vi "Sub_vi_ejecutar_Edificio_3.vi"(0 "Edificio_string":string, 1 "Serv_Numeric":u8, 2 "De":u8=1 min=1 max=16, 3 "Hasta":u8=16 min=1 max=16, 4 "edo_actual_aula":bool, 5 "rango":bool, 6 "+                 -":bool) -> ()   [LabVIEW 2017]
uses:
  GlobalFag.vi
  Global_comSerie.vi
  <vilib>/Instr/_visa.llb/VISA Configure Serial Port (Instr).vi
panel:
  in  "x":u8
  out "sh_reg2":u8
  out "sh_reg":u8
  in  "act_vac":bool
  out "estado 2":bool[](array[boolean])
  out "aula_fin":u8
  in  "stop_edificio":bool
  in  "Servicios":bool[](array[boolean])
  # "+/- Edo. Actual"
  # "Conf para Edif A, aula 15"
  # "Servicio"
  # "Aplicar a un rango"
  # "Luz"
  # "Aire"
  # "Proyector"
  # "Agua"
  # "Acceso"
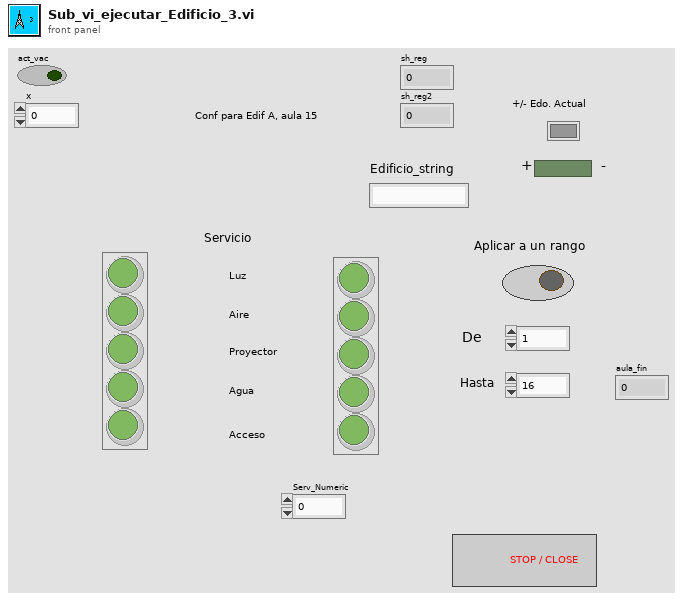
[diagram p1: front panel]
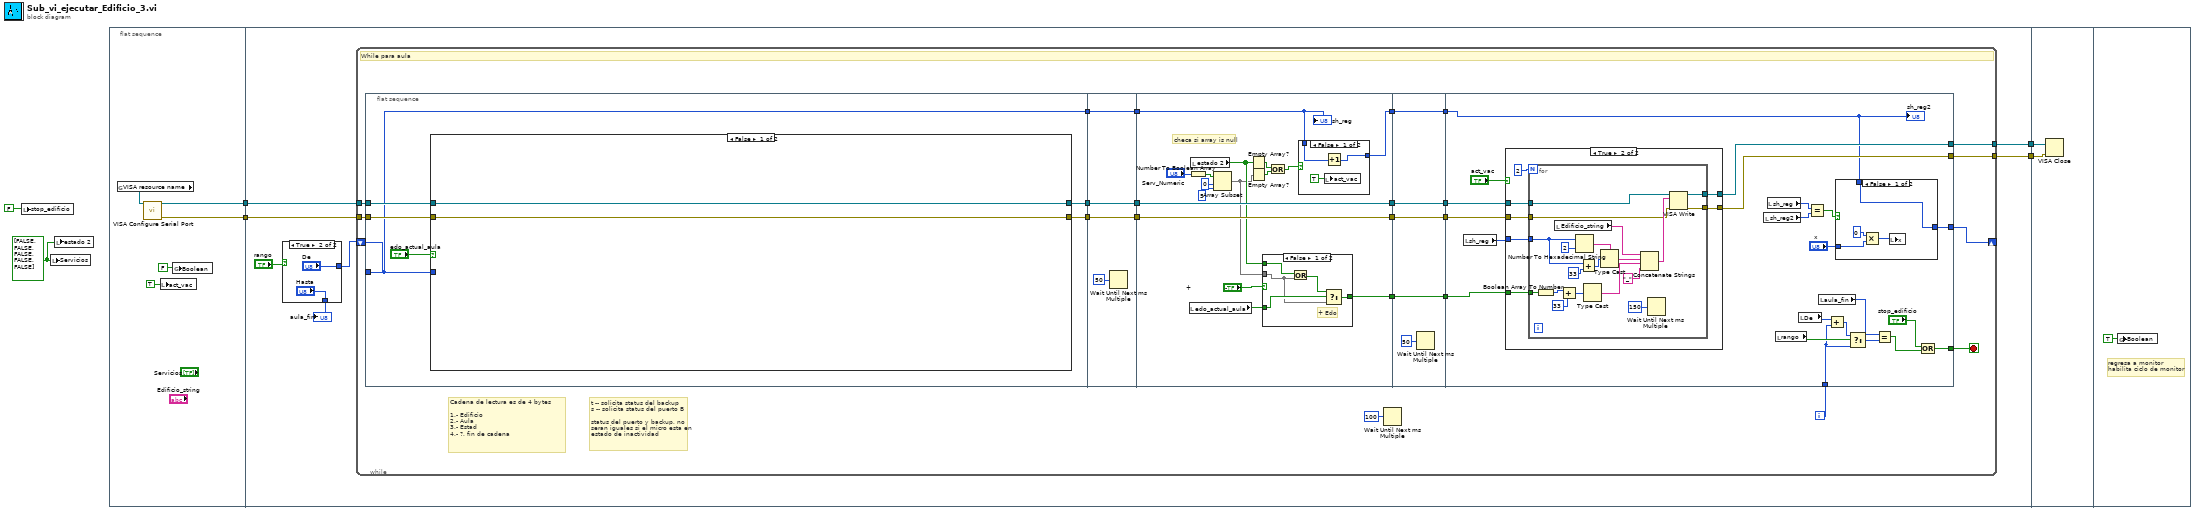
[diagram p0: block diagram]
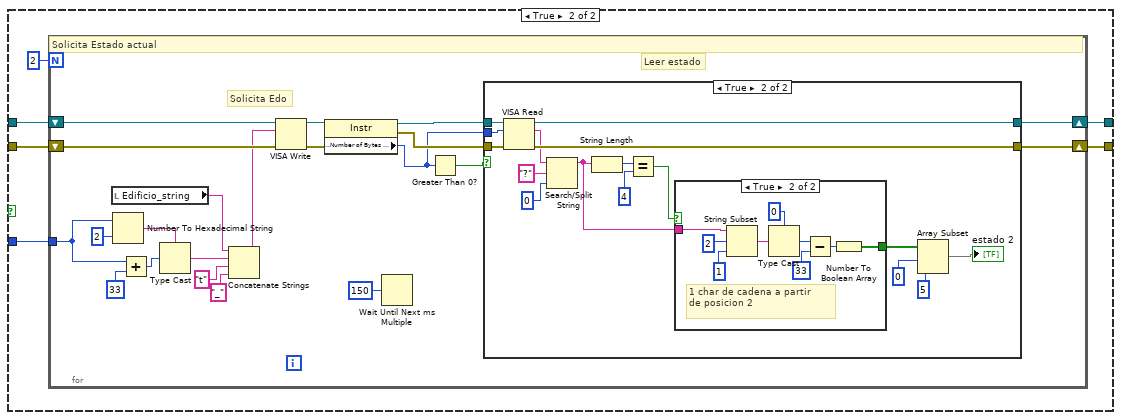
[diagram p2: hidden frame]
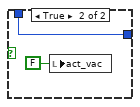
[diagram p5: hidden frame]
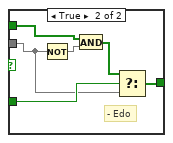
[diagram p6: hidden frame]
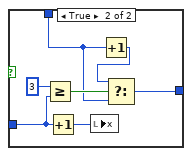
[diagram p7: hidden frame]
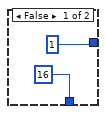
[diagram p9: hidden frame]
diagram:
  w1 = bool[] [FALSE, FALSE, FALSE, FALSE, FALSE] ("Servicios")
  n1 = local write "stop_edificio"(FALSE ("Loading")) -> ()
  n2 = local write "Servicios"(w1) -> ()
  n3 = local write "estado 2"(w1) -> ()
  n4 = flat-sequence {
    tunnel: [w11] -> w5
    tunnel: [w10] -> w4
    tunnel: w4 -> [w15]
    tunnel: w5 -> [w16]
    tunnel: [w13] -> w3
    tunnel: [w12] -> w2
    tunnel: w3 -> [w211]
    tunnel: w2 -> [w210]
    frame #0 {
      n5 = global read "Global_comSerie.vi" "VISA resource name"() -> (w8:refnum<visa-resource-name>)
      n6 = call-poly "VISA Configure Serial Port"("VISA resource name"=w8) -> ("VISA resource name out"=w11:refnum<visa-resource-name>, "error out"=w10:errorcluster)  [unwired: 13 in]
      n7 = local write "act_vac"(TRUE ("act_vac")) -> ()
      n8 = global write "GlobalFag.vi" "Boolean"(FALSE ("Boolean")) -> ()
    }
    frame #1 {
      n9 = case shown="True" "rango" {
        tunnel: [u8 1 ("width (-)") "De"] -> w14
        tunnel: [u8 16 ("width (-)") "Hasta"] -> w17
        frame False {
        }
        frame True {
        }
      }
      "aula_fin" <- w17
      n10 = while {
        shift-right: [w21] -> _
        shift-left: w14 -> [w40]
        tunnel: w16 -> [w39]
        tunnel: w15 -> [w38]
        tunnel: [w23] -> w13
        tunnel: [w22] -> w12
        i -> [w19]
        stop <- w20 stop-if-true
        # "Cadena de lectura es de 4 bytes\n\n1.- Edificio\n2.- Aula\n3.- Estad\n4.- ?, fin de cadena"
        # "t -- solicita status del backup\ns -- solicita status del puerto B\n\nstatus del puerto y backup, no \nseran iguales si el micro esta en\nestado de inactividad"
        # "While para aula"
        n11 = flat-sequence {
          tunnel: w40 -> [w44]
          tunnel: w39 -> [w46]
          tunnel: w38 -> [w45]
          tunnel: [w44] -> w37
          tunnel: [w43] -> w35
          tunnel: [w42] -> w33
          tunnel: w37 -> [w107]
          tunnel: [w107] -> w36
          tunnel: w35 -> [w106]
          tunnel: [w106] -> w34
          tunnel: w33 -> [w105]
          tunnel: [w105] -> w32
          tunnel: [w112] -> w31
          tunnel: w36 -> [w111]
          tunnel: [w122] -> w29
          tunnel: [w121] -> w27
          tunnel: w34 -> [w121]
          tunnel: [w120] -> w25
          tunnel: w32 -> [w120]
          tunnel: w31 -> [w144]
          tunnel: [w144] -> w30
          tunnel: w29 -> [w143]
          tunnel: [w143] -> w28
          tunnel: w27 -> [w142]
          tunnel: [w142] -> w26
          tunnel: w25 -> [w141]
          tunnel: [w141] -> w24
          tunnel: w30 -> [w155]
          tunnel: w28 -> [w164]
          tunnel: w26 -> [w166]
          tunnel: w24 -> [w165]
          tunnel: [w161] -> w23
          tunnel: [w160] -> w22
          tunnel: [w154] -> w21
          tunnel: [w146] -> w20
          tunnel: w19 -> [w145]
          frame #0 {
            n12 = case shown="False" "edo_actual_aula" {
              tunnel: w44 -> [_ w54]
              tunnel: w46 -> [w49 w53]
              tunnel: w45 -> [w48 w52]
              tunnel: [w49 w51] -> w43
              tunnel: [w48 w50] -> w42
              frame False {
              }
              frame True {
                n13 = for {
                  N: 2 -> [_]
                  tunnel: w54 -> [w58]
                  shift-right: [w74] -> w51
                  shift-left: w53 -> [w72]
                  shift-right: [w73] -> w50
                  shift-left: w52 -> [w71]
                  # "Solicita Edo"
                  # "Leer estado"
                  # "Solicita Estado actual"
                  n14 = local read "Edificio_string"() -> (w56:string)
                  n15 = Number To Hexadecimal String(1:u8 2 ("width (-)"), 2:w58) -> (0:w60:string)
                  n16 = Add(x=w58, y=u8 33 ("width (-)")) -> (x+y=w62:u8)
                  n17 = Type Cast(type=w60, x=w62) -> (*(type *) &x=w57:string)
                  n18 = Concatenate Strings(w56, w57, "t" ("string"), "_" ("string")) -> (w70:string)
                  n19 = VISA Write(VISA resource name=w72, write buffer=w70, error in (no error)=w71) -> (VISA resource name out=w75:refnum<visa-resource-name>, error out=w76:errorcluster)  [unwired: 1 out]
                  n20 = property class="Instr"(reference=w75, error in=w76) -> (reference out=w65:refnum<visa-resource-name>, error out=w64:errorcluster, "Serial Settings:Number of Bytes at Serial Port"=w63:u32)
                  n21 = Wait Until Next ms Multiple(millisecond multiple=u32 150) -> ()  [unwired: 1 out]
                  n22 = Greater Than 0?(x=w63) -> (x > 0?=w66:bool)
                  n23 = case shown="True" w66 {
                    tunnel: w65 -> [w77 w94]
                    tunnel: w64 -> [w78 w93]
                    tunnel: [w78 w92] -> w73
                    tunnel: [w77 w91] -> w74
                    tunnel: w63 -> [_ w90]
                    frame False {
                    }
                    frame True {
                      n24 = VISA Read(VISA resource name=w94, byte count=w90, error in (no error)=w93) -> (VISA resource name out=w91:refnum<visa-resource-name>, read buffer=w86:string, error out=w92:errorcluster)  [unwired: 1 out]
                      n25 = Search/Split String(string=w86, search string/char (-)="?", offset (0)=u8 0) -> (substring before match=w84:string)  [unwired: 2 out]
                      n26 = String Length(string=w84) -> (length=w89:i32)
                      n27 = Equal?(x=w89, y=4) -> (x = y?=w85:bool)
                      n28 = case shown="True" w85 {
                        tunnel: w84 -> [_ w96]
                        tunnel: [_ w95] -> w81
                        frame False {
                        }
                        frame True {
                          # "1 char de cadena a partir \nde posicion 2"
                          n29 = String Subset(string=w96, offset (0)=2, length (rest)=1 ("length (rest)")) -> (substring=w100:string)
                          n30 = Type Cast(type=u8 0 ("width (-)"), x=w100) -> (*(type *) &x=w98:u8)
                          n31 = Subtract(x=w98, y=u8 33) -> (x-y=w99:u8)
                          n32 = Number To Boolean Array(number=w99) -> (Boolean array=w95:bool[])
                        }
                      }
                      n33 = Array Subset(array=w81, index=0, length=5) -> (→"estado 2":bool[])
                    }
                  }
                }
              }
            }
          }
          frame #1 {
            n34 = Wait Until Next ms Multiple(millisecond multiple=u32 50) -> ()  [unwired: 1 out]
          }
          frame #2 {
            # "checa si array is null"
            n35 = local read "edo_actual_aula"() -> (w119:bool)
            n36 = Number To Boolean Array(number="Serv_Numeric") -> (Boolean array=w116:bool[])
            n37 = local read "estado 2"() -> (w110:bool[])
            n38 = Array Subset(array=w116, index=0, length=5) -> (w109:bool[])
            n39 = Empty Array?(array=w110) -> (empty?=w115:bool)
            n40 = Empty Array?(array=w109) -> (empty?=w114:bool)
            n41 = case shown="False" "+                 -" {
              tunnel: [w133 w139] -> w122
              tunnel: w119 -> [w131 w136]
              tunnel: w110 -> [w130 w135]
              tunnel: w109 -> [w129 w134]
              frame False {
                # "+ Edo"
                n42 = Or(x=w130, y=w129) -> (x .or. y?=w132:bool[])
                n43 = Select(t=w132, s=w131, f=w129) -> (s? t:f=w133:bool[])
              }
              frame True {
                # "- Edo"
                n44 = Not(x=w134) -> (.not. x?=w138:bool[])
                n45 = And(x=w135, y=w138) -> (x .and. y?=w137:bool[])
                n46 = Select(t=w137, s=w136, f=w134) -> (s? t:f=w139:bool[])
              }
            }
            n47 = Or(x=w115, y=w114) -> (x .or. y?=w113:bool)
            n48 = case shown="False" w113 {
              tunnel: [w125 w127] -> w112
              tunnel: w111 -> [w126 w127]
              frame False {
                n49 = local write "act_vac"(TRUE ("act_vac")) -> ()
                n50 = Increment(x=w126) -> (x+1=w125:u8)
              }
              frame True {
                n51 = local write "act_vac"(FALSE ("act_vac")) -> ()
              }
            }
            "sh_reg" <- w111
          }
          frame #3 {
            n52 = Wait Until Next ms Multiple(millisecond multiple=u32 50) -> ()  [unwired: 1 out]
          }
          frame #4 {
            n53 = local read "sh_reg"() -> (w162:u8)
            n54 = case shown="True" "act_vac" {
              tunnel: [w179 w186] -> w160
              tunnel: [w178 w185] -> w161
              tunnel: w162 -> [_ w184]
              tunnel: w166 -> [w178 w182]
              tunnel: w165 -> [w179 w181]
              tunnel: w164 -> [_ w180]
              frame False {
              }
              frame True {
                n55 = for {
                  N: 2 -> [_]
                  tunnel: [w194] -> w186
                  tunnel: [w193] -> w185
                  tunnel: w184 -> [w191]
                  tunnel: w180 -> [w190]
                  tunnel: w182 -> [w189]
                  tunnel: w181 -> [w188]
                  n56 = Boolean Array To Number(Boolean array=w190) -> (number=w192:u8)
                  n57 = local read "Edificio_string"() -> (w205:string)
                  n58 = Add(x=w192, y=u8 33) -> (x+y=w203:u8)
                  n59 = Number To Hexadecimal String(1:u8 2 ("width (-)"), 2:w191) -> (0:w200:string)
                  n60 = Add(x=w191, y=u8 33 ("width (-)")) -> (x+y=w202:u8)
                  n61 = Type Cast(x=w203) -> (*(type *) &x=w204:string)  [unwired: 1 in]
                  n62 = Type Cast(type=w200, x=w202) -> (*(type *) &x=w199:string)
                  n63 = Concatenate Strings(w205, w199, w204, "_" ("string")) -> (w201:string)
                  n64 = Wait Until Next ms Multiple(millisecond multiple=u32 150) -> ()  [unwired: 1 out]
                  n65 = VISA Write(VISA resource name=w189, write buffer=w201, error in (no error)=w188) -> (VISA resource name out=w193:refnum<visa-resource-name>, error out=w194:errorcluster)  [unwired: 1 out]
                }
              }
            }
            n66 = local read "sh_reg2"() -> (w158:u8)
            n67 = local read "sh_reg"() -> (w159:u8)
            n68 = local read "rango"() -> (w150:bool)
            n69 = local read "De"() -> (w152:u8)
            n70 = Equal?(x=w159, y=w158) -> (x = y?=w157:bool)
            n71 = local read "aula_fin"() -> (w149:u8)
            n72 = Add(x=w152, y=w145) -> (x+y=w151:i32)
            n73 = case shown="False" w157 {
              tunnel: "x" -> [w170 w176]
              tunnel: w155 -> [w167 w173]
              tunnel: [w167 w171] -> w154
              frame False {
                n74 = Multiply(x=u8 0, y=w170) -> (x*y=w168:u8)
                n75 = local write "x"(w168) -> ()
              }
              frame True {
                n76 = Greater Or Equal?(x=u8 3, y=w176) -> (x >= y?=w174:bool)
                n77 = Increment(x=w176) -> (x+1=w175:u8)
                n78 = local write "x"(w175) -> ()
                n79 = Increment(x=w173) -> (x+1=w172:u8)
                n80 = Select(t=w172, s=w174, f=w173) -> (s? t:f=w171:u8)
              }
            }
            n81 = Select(t=w151, s=w150, f=w145) -> (s? t:f=w153:i32)
            n82 = Equal?(x=w149, y=w153) -> (x = y?=w147:bool)
            n83 = Compound Arithmetic op=OR("stop_edificio", w147) -> (w146:bool)
            "sh_reg2" <- w155
          }
        }
        n84 = Wait Until Next ms Multiple(millisecond multiple=u32 100) -> ()  [unwired: 1 out]
      }
    }
    frame #2 {
      n85 = VISA Close(VISA resource name=w211, error in (no error)=w210) -> ()  [unwired: 1 out]
    }
    frame #3 {
      # "regresa a monitor\nhabilita ciclo de monitor"
      n86 = global write "GlobalFag.vi" "Boolean"(TRUE ("Boolean")) -> ()
    }
  }
